vi "7.7.4-UDP-Forbrain_to_OCU-Client.vi"() -> ()   [LabVIEW 2010]
doc: "This VI implements a client for the Named Service UDP Server.vi.\nIt connects to a service by specifying the server address and the name of the service. After sending a 'Hello' string to the server, the client receives the string sent by the server, displays the string and closes the connection.\n\n<b>Note:</b> This VI is built to work with the Named Service UDP Server.vi in UDP.llb."
uses:
  6-OCU Neurons/CommonIndicators.ctl
  7.0-Global.vi
panel:
  out "Main Indicators":T1={"Speed"=0.0, " Heading"={0.0, 34.390870865624734}, "MissionTime"=0.0, "Battery"=0.0, "MAP"=FALSE, "LIDAR"=FALSE, "ManualMissionMap"=bytes[0], "ManualModeLIDAR"=bytes[0], "ManualModeStop"=FALSE, "How?"=FALSE, "Where?"=FALSE, "What?"=FALSE, "ActManual"=FALSE, "CollisionLight "=FALSE, "Ready"=FALSE} {"Battery" scale=16.0..24.0; "MissionTime" scale=0.0..10.0; "Heading" scale=180.0..-180.0; "Speed" scale=0.0..4.0}
  out "String":string
  out "error out":errorcluster
  in  "error in":errorcluster
  # "Instructions:\n1. Open Named Service UDP Server.vi located in the same library.\n2. Follow the instructions on it's front panel.\n\nNote: This VI is built to work with the Named Service UDP Server.vi in UDP.llb."
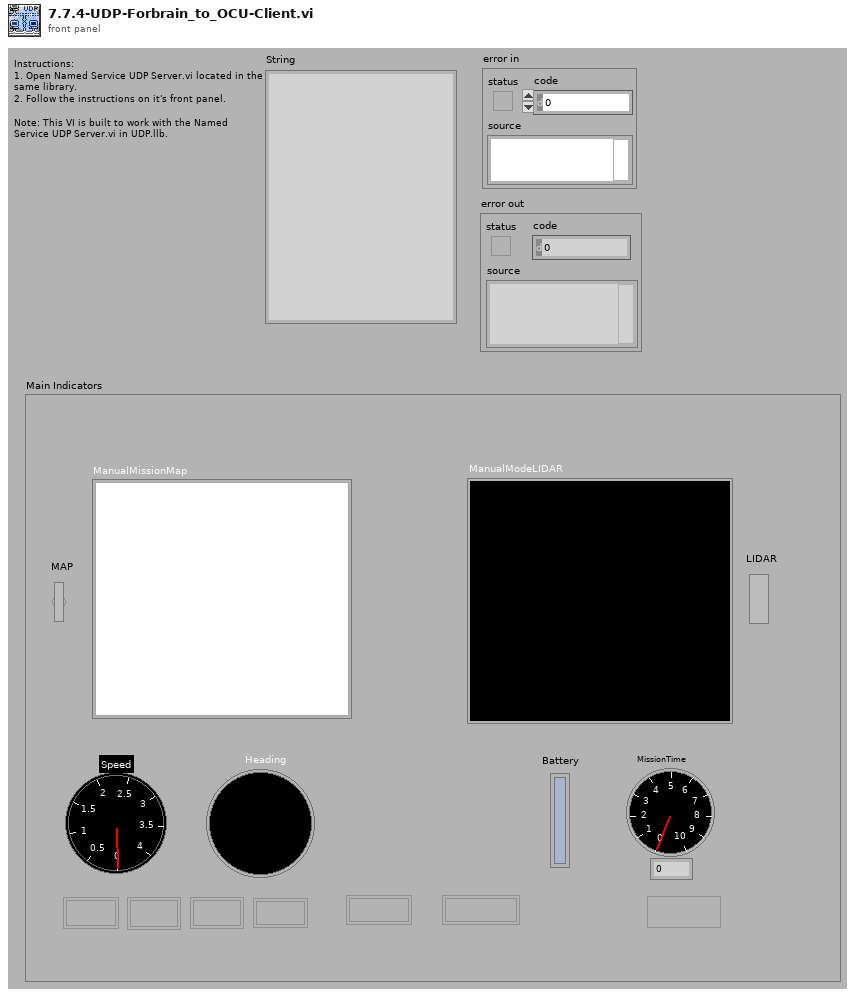
[diagram p1: front panel]
types:
  T1 = typedef "CommonIndicators.ctl" = cluster{"Speed":dbl, " Heading":cluster{dbl, dbl}, "MissionTime":dbl, "Battery":dbl, "MAP":bool, "LIDAR":bool, "ManualMissionMap":picture, "ManualModeLIDAR":picture, "ManualModeStop":bool, "How?":bool, "Where?":bool, "What?":bool, "ActManual":bool, "CollisionLight ":bool, "Ready":bool}
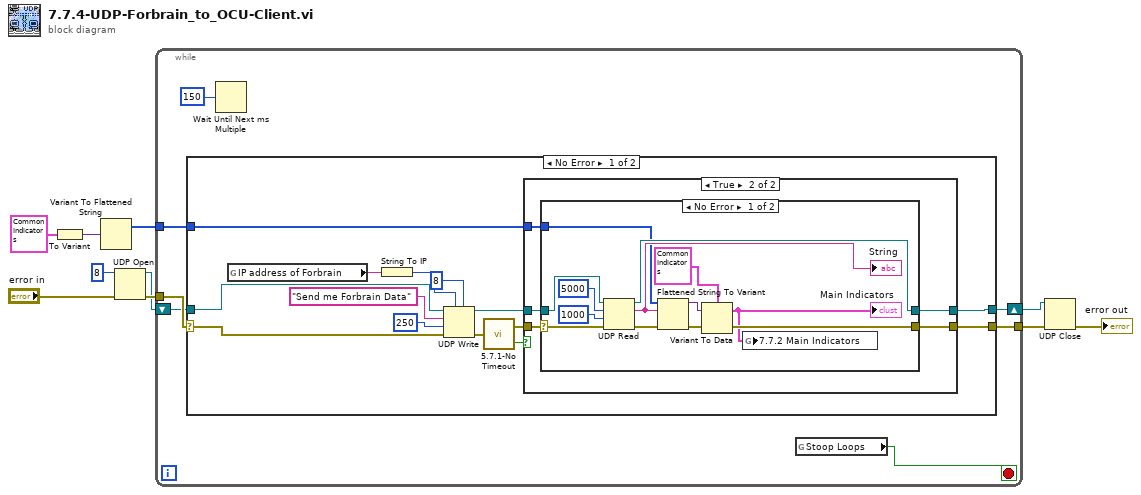
[diagram p0: block diagram]
diagram:
  n1 = To Variant(anything=T1 {"Speed"=0.0, " Heading"={0.0, 34.390870865624734}, "MissionTime"=0.0, "Battery"=0.0, "MAP"=FALSE, "LIDAR"=FALSE, "ManualMissionMap"=bytes[0], "ManualModeLIDAR"=bytes[0], "ManualModeStop"=FALSE, "How?"=FALSE, "Where?"=FALSE, "What?"=FALSE, "ActManual"=FALSE, "CollisionLight "=FALSE, "Ready"=FALSE} ("data")) -> (Variant=w3:variant)
  n2 = Variant To Flattened String(Variant=w3) -> (1:w2:i16[])  [unwired: 1 out]
  n3 = UDP Open(8:"error in", 11:u16 8) -> (port=w7:refnum<k16>, 0:w8:errorcluster)  [unwired: 3 in, 1 out]
  n4 = while {
    tunnel: [w17] -> w5
    tunnel: w8 -> [w16]
    shift-right: [w14] -> w6
    shift-left: w7 -> [w15]
    tunnel: w2 -> [w12]
    stop <- w11 stop-if-true
    n5 = case shown="No Error" w16 {
      selector: w16 -> [w31 w55]
      tunnel: [w26 w55] -> w17
      tunnel: w15 -> [w30 w54]
      tunnel: [w25 w54] -> w14
      tunnel: w12 -> [w20 _]
      frame No Error {
        n6 = global read "7.0-Global.vi" "IP address of Forbrain"() -> (w19:string)
        n7 = String To IP(1:w19) -> (0:w29:u32)
        n8 = UDP Write(address=w29, port or service name=u16 8, connection ID=w30, data in="Send me Forbrain Data", 8:w31, 9:250 ("timeout ms (25000)")) -> (error out=w24:errorcluster, 3:w27:refnum<k16>)
        n9 = call "5.7.1-No Timeout.vi"("error in (no error)"=w24) -> ("No Timeout"=w22:bool, "error out"=w23:errorcluster)
        n10 = case shown="True" w22 {
          tunnel: w23 -> [w33 w38]
          tunnel: w27 -> [w32 w37]
          tunnel: [w32 w36] -> w25
          tunnel: [w33 w35] -> w26
          tunnel: w20 -> [_ w34]
          frame False {
          }
          frame True {
            n11 = case shown="No Error" w38 {
              selector: w38 -> [w51 w52]
              tunnel: w37 -> [w50 w53]
              tunnel: [w48 w53] -> w36
              tunnel: [w41 w52] -> w35
              tunnel: w34 -> [w45 _]
              frame No Error {
                n12 = UDP Read(connection ID=w50, max size (548)=5000, timeout ms (25000)=1000, 8:w51) -> (data out=w46:string, error out=w42:errorcluster, 3:w48:refnum<k16>)  [unwired: 2 out]
                "String" <- w46
                n13 = Flattened String To Variant(4:w42, 6:w46, 7:w45) -> (0:w43:errorcluster, 3:w44:variant)
                n14 = Variant To Data(error in=w43, Variant=w44, type=T1 {"Speed"=0.0, " Heading"={0.0, 34.390870865624734}, "MissionTime"=0.0, "Battery"=0.0, "MAP"=FALSE, "LIDAR"=FALSE, "ManualMissionMap"=bytes[0], "ManualModeLIDAR"=bytes[0], "ManualModeStop"=FALSE, "How?"=FALSE, "Where?"=FALSE, "What?"=FALSE, "ActManual"=FALSE, "CollisionLight "=FALSE, "Ready"=FALSE} ("data")) -> (error out=w41:errorcluster, data=w40:T1)
                "Main Indicators" <- w40
                n15 = global write "7.0-Global.vi" "7.7.2 Main Indicators"(w40) -> ()
              }
              frame Error {
              }
            }
          }
        }
      }
      frame Error {
      }
    }
    n16 = Wait Until Next ms Multiple(millisecond multiple=u32 150) -> ()  [unwired: 1 out]
    n17 = global read "7.0-Global.vi" "Stoop Loops"() -> (w11:bool)
  }
  n18 = UDP Close(connection ID=w6, 8:w5) -> (error out=→"error out":errorcluster)  [unwired: 1 out]
